vi "VI Tree.vi"   [LabVIEW 2015, in "Zaber A Series.lvlib"]
doc: "This is the instrument driver for the Zaber ASCII Protocol. The VI Tree displays all the user-callable VIs of the instrument driver in an organized table."
uses:
  Zaber A Series.lvlib
  Configure/Virtual Axis/Set Virtual Axis Speed.vi
  Action-Status/Streaming/Stream Line.vi
  Action-Status/Lockstep/Lockstep Move (FW7).vi
  Action-Status/Streaming/Open Stream.vi
  Action-Status/Streaming/Set Stream Speed and Acceleration.vi
  Action-Status/Lockstep/Lockstep Move at Velocity.vi
  Action-Status/Virtual Axis/Virtual Axis Move.vi
  Action-Status/Virtual Axis/Virtual Axis Move at Velocity.vi
  Configure/Virtual Axis/Create Virtual Axis (by Angle).vi
  Action-Status/Streaming/Stream Circle.vi
  Action-Status/Streaming/Stream Arc.vi
  Action-Status/Streaming/Stream Wait for Input (Analog).vi
  Utility/Low Level/Convert Device Units to Speed Units.vi
  Utility/Low Level/Convert Device Units to Position Units.vi
panel:
  # "(c) 2017-2021 Zaber Technologies.  ALL RIGHTS RESERVED."
  # "SEE DIAGRAM\nFOR VI TREE."
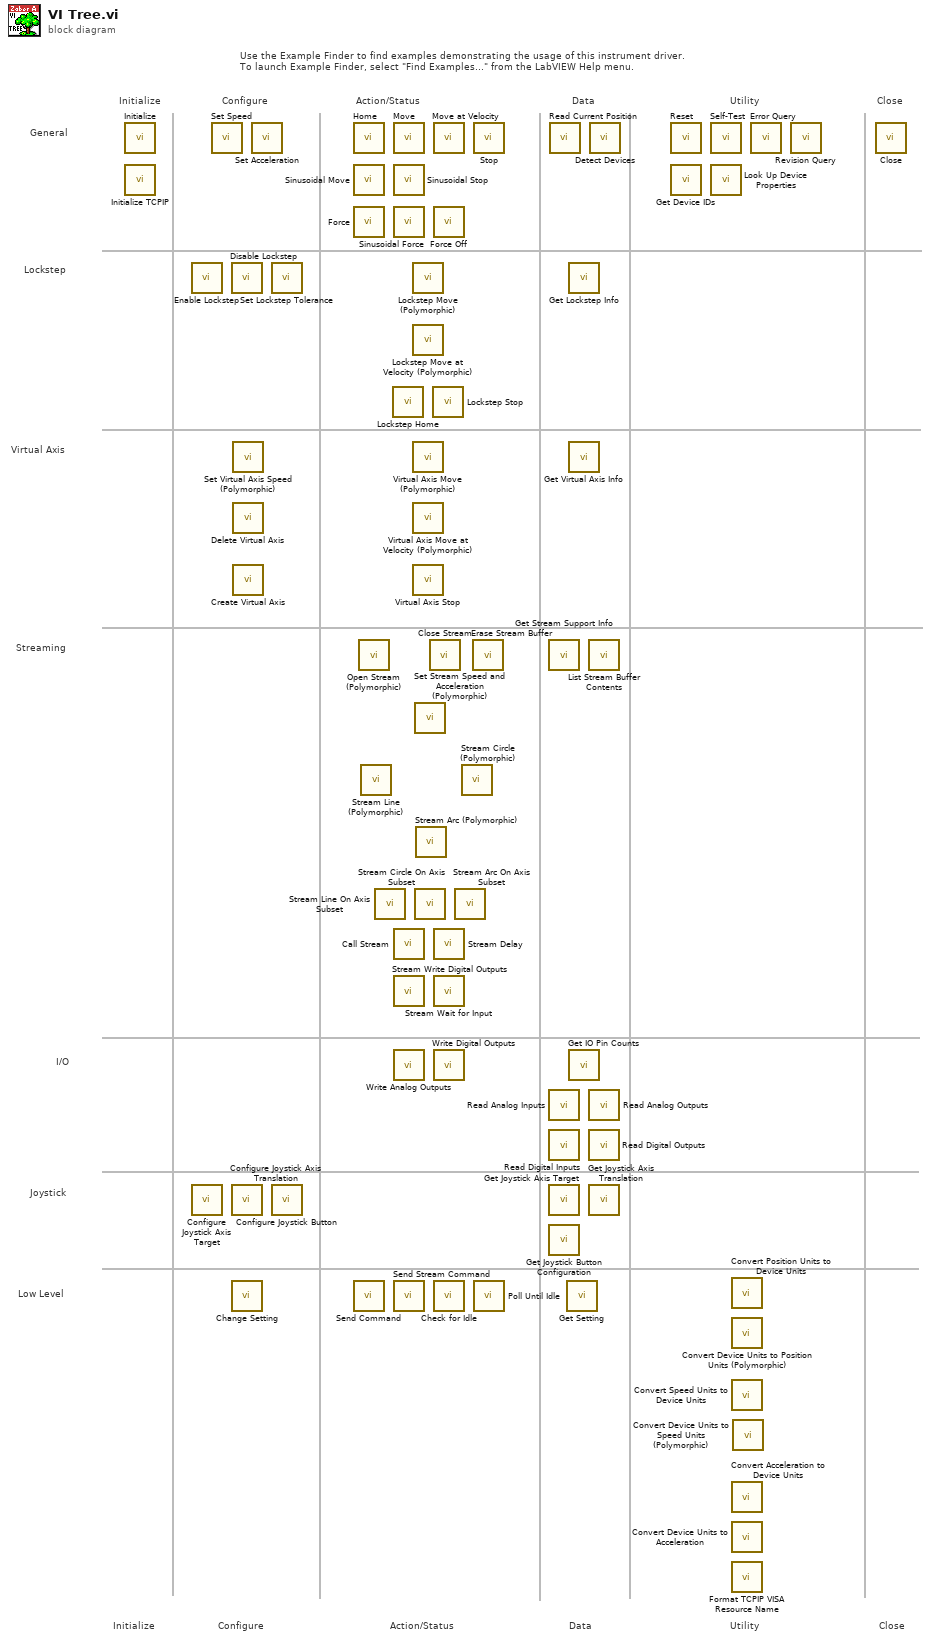
[diagram p0: block diagram]
diagram:
  # "Configure"
  # "Data"
  # "Utility"
  # "Action/Status"
  # "Close"
  # "Initialize"
  # "Joystick"
  # "Streaming"
  # "Virtual Axis"
  # "General"
  # "Lockstep"
  # "I/O"
  # "Low Level"
  # "Configure"
  # "Data"
  # "Use the Example Finder to find examples demonstrating the usage of this instrument driver.\nTo launch Example Finder, select \"Find Examples...\" from the LabVIEW Help menu."
  # "Utility"
  # "Action/Status"
  # "Close"
  # "Initialize"
  n1 = call "Initialize.vi"() -> ()  [unwired: 10 in, 2 out]
  n2 = call "Initialize TCPIP.vi"() -> ()  [unwired: 10 in, 2 out]
  n3 = call "Enable Lockstep.vi"() -> ()  [unwired: 10 in, 2 out]
  n4 = call "Configure Joystick Axis Target.vi"() -> ()  [unwired: 10 in, 2 out]
  n5 = call "Set Speed.vi"() -> ()  [unwired: 10 in, 2 out]
  n6 = call "Disable Lockstep.vi"() -> ()  [unwired: 10 in, 2 out]
  n7 = call "Configure Joystick Axis Translation.vi"() -> ()  [unwired: 10 in, 2 out]
  n8 = call "Change Setting.vi"() -> ()  [unwired: 10 in, 2 out]
  n9 = call-poly "Set Virtual Axis Speed (Polymorphic).vi"() -> ()  [unwired: 10 in, 2 out]
  n10 = call "Delete Virtual Axis.vi"() -> ()  [unwired: 10 in, 2 out]
  n11 = call-poly "Create Virtual Axis.vi"() -> ()  [unwired: 10 in, 2 out]
  n12 = call "Set Acceleration.vi"() -> ()  [unwired: 10 in, 2 out]
  n13 = call "Set Lockstep Tolerance.vi"() -> ()  [unwired: 10 in, 2 out]
  n14 = call "Configure Joystick Button.vi"() -> ()  [unwired: 10 in, 2 out]
  n15 = call "Home.vi"() -> ()  [unwired: 10 in, 2 out]
  n16 = call "Sinusoidal Move.vi"() -> ()  [unwired: 10 in, 2 out]
  n17 = call "Force.vi"() -> ()  [unwired: 10 in, 2 out]
  n18 = call "Send Command.vi"() -> ()  [unwired: 6 in, 6 out]
  n19 = call-poly "Open Stream (Polymorphic).vi"() -> ()  [unwired: 10 in, 2 out]
  n20 = call-poly "Stream Line (Polymorphic).vi"() -> ()  [unwired: 10 in, 2 out]
  n21 = call "Stream Line On Axis Subset.vi"() -> ()  [unwired: 10 in, 2 out]
  n22 = call "Lockstep Home.vi"() -> ()  [unwired: 10 in, 2 out]
  n23 = call "Move.vi"() -> ()  [unwired: 10 in, 2 out]
  n24 = call "Sinusoidal Stop.vi"() -> ()  [unwired: 10 in, 2 out]
  n25 = call "Sinusoidal Force.vi"() -> ()  [unwired: 10 in, 2 out]
  n26 = call "Call Stream.vi"() -> ()  [unwired: 10 in, 2 out]
  n27 = call "Stream Write Digital Outputs.vi"() -> ()  [unwired: 10 in, 2 out]
  n28 = call "Write Analog Outputs.vi"() -> ()  [unwired: 10 in, 2 out]
  n29 = call "Send Stream Command.vi"() -> ()  [unwired: 10 in, 2 out]
  n30 = call-poly "Lockstep Move (Polymorphic).vi"() -> ()  [unwired: 10 in, 2 out]
  n31 = call-poly "Lockstep Move at Velocity (Polymorphic).vi"() -> ()  [unwired: 10 in, 2 out]
  n32 = call-poly "Virtual Axis Move (Polymorphic).vi"() -> ()  [unwired: 10 in, 2 out]
  n33 = call-poly "Virtual Axis Move at Velocity (Polymorphic).vi"() -> ()  [unwired: 10 in, 2 out]
  n34 = call "Virtual Axis Stop.vi"() -> ()  [unwired: 10 in, 2 out]
  n35 = call-poly "Set Stream Speed and Acceleration (Polymorphic).vi"() -> ()  [unwired: 10 in, 2 out]
  n36 = call "Stream Circle On Axis Subset.vi"() -> ()  [unwired: 10 in, 2 out]
  n37 = call-poly "Stream Arc (Polymorphic).vi"() -> ()  [unwired: 10 in, 2 out]
  n38 = call "Close Stream.vi"() -> ()  [unwired: 10 in, 2 out]
  n39 = call "Lockstep Stop.vi"() -> ()  [unwired: 10 in, 2 out]
  n40 = call "Move at Velocity.vi"() -> ()  [unwired: 10 in, 2 out]
  n41 = call "Force Off.vi"() -> ()  [unwired: 10 in, 2 out]
  n42 = call "Stream Delay.vi"() -> ()  [unwired: 10 in, 2 out]
  n43 = call-poly "Stream Wait for Input.vi"() -> ()  [unwired: 10 in, 2 out]
  n44 = call "Write Digital Outputs.vi"() -> ()  [unwired: 10 in, 2 out]
  n45 = call "Check for Idle.vi"() -> ()  [unwired: 9 in, 3 out]
  n46 = call "Stream Arc On Axis Subset.vi"() -> ()  [unwired: 14 in, 2 out]
  n47 = call-poly "Stream Circle (Polymorphic).vi"() -> ()  [unwired: 10 in, 2 out]
  n48 = call "Erase Stream Buffer.vi"() -> ()  [unwired: 10 in, 2 out]
  n49 = call "Stop.vi"() -> ()  [unwired: 10 in, 2 out]
  n50 = call "Poll Until Idle.vi"() -> ()  [unwired: 10 in, 2 out]
  n51 = call "Get Stream Support Info.vi"() -> ()  [unwired: 8 in, 4 out]
  n52 = call "Read Analog Inputs.vi"() -> ()  [unwired: 9 in, 3 out]
  n53 = call "Read Digital Inputs.vi"() -> ()  [unwired: 9 in, 3 out]
  n54 = call "Get Joystick Axis Target.vi"() -> ()  [unwired: 7 in, 5 out]
  n55 = call "Get Joystick Button Configuration.vi"() -> ()  [unwired: 9 in, 3 out]
  n56 = call "Read Current Position.vi"() -> ()  [unwired: 9 in, 3 out]
  n57 = call "Get Setting.vi"() -> ()  [unwired: 6 in, 6 out]
  n58 = call "Get Lockstep Info.vi"() -> ()  [unwired: 7 in, 5 out]
  n59 = call "Get Virtual Axis Info.vi"() -> ()  [unwired: 6 in, 6 out]
  n60 = call "Get IO Pin Counts.vi"() -> ()  [unwired: 6 in, 6 out]
  n61 = call "List Stream Buffer Contents.vi"() -> ()  [unwired: 9 in, 3 out]
  n62 = call "Read Analog Outputs.vi"() -> ()  [unwired: 9 in, 3 out]
  n63 = call "Read Digital Outputs.vi"() -> ()  [unwired: 9 in, 3 out]
  n64 = call "Get Joystick Axis Translation.vi"() -> ()  [unwired: 6 in, 6 out]
  n65 = call "Detect Devices.vi"() -> ()  [unwired: 8 in, 4 out]
  n66 = call "Reset.vi"() -> ()  [unwired: 10 in, 2 out]
  n67 = call "Get Device IDs.vi"() -> ()  [unwired: 8 in, 4 out]
  n68 = call "Self-Test.vi"() -> ()  [unwired: 9 in, 3 out]
  n69 = call "Look Up Device Properties.vi"() -> ()  [unwired: 8 in, 4 out]
  n70 = call "Convert Position Units to Device Units.vi"() -> ()  [unwired: 9 in, 3 out]
  n71 = call-poly "Convert Device Units to Position Units (Polymorphic).vi"() -> ()  [unwired: 11 in, 1 out]
  n72 = call "Convert Speed Units to Device Units.vi"() -> ()  [unwired: 9 in, 3 out]
  n73 = call "Convert Acceleration to Device Units.vi"() -> ()  [unwired: 9 in, 3 out]
  n74 = call "Convert Device Units to Acceleration.vi"() -> ()  [unwired: 11 in, 1 out]
  n75 = call "Format TCPIP VISA Resource Name.vi"() -> ()  [unwired: 11 in, 1 out]
  n76 = call-poly "Convert Device Units to Speed Units (Polymorphic).vi"() -> ()  [unwired: 11 in, 1 out]
  n77 = call "Error Query.vi"() -> ()  [unwired: 8 in, 4 out]
  n78 = call "Revision Query.vi"() -> ()  [unwired: 8 in, 4 out]
  n79 = call "Close.vi"() -> ()  [unwired: 11 in, 1 out]
